vi "Agilent PWM Trigger and Fetch.vi"(7 "Agilent PWM":T1, 8 "error in (no error)":errorcluster, 10 "Timeout (10000ms)":u32=10000, 11 "VISA Resource Name":refnum<visa-resource-name>) -> (0 "error out":errorcluster, 2 "Data Reading":T2 caption="This reading is allways in the base units\ni.e. V, A, Ohms, Hz, Sec, dB, etc." format="%#_10f", 3 "dup VISA Resource Name":refnum<visa-resource-name>)   [LabVIEW 2011]
doc: "This VI for the HP 8753 is used to read the sweep type.\n\n0 LINEAR FREQ\n1 LOG FREQ\n2 LIST FREQ\n3 CW TIME\n4 POWER SWEEP"
uses:
  PWM Measurement.ctl
  TypeDefs/Agilent PWM Instrument Info.ctl
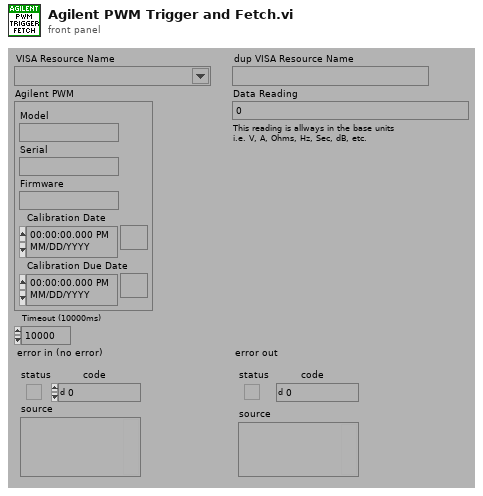
[diagram p1: front panel]
types:
  T1 = typedef "Agilent PWM Instrument Info.ctl" = cluster{"Model":string, "Serial":string, "Firmware":string, "Calibration Date":timestamp, "Calibration Due Date":timestamp}
  T2 = typedef "PWM Measurement.ctl" = dbl
  T3 = typedef "Agilent PWM Model.ctl" = enum16{"Not Supported", "E4418X", "E4419X", "U2000X"}
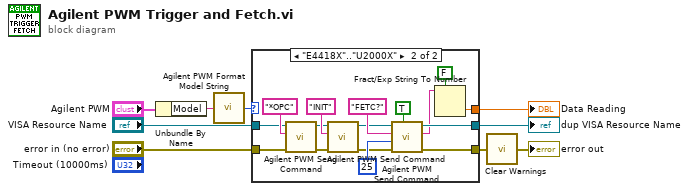
[diagram p0: block diagram]
diagram:
  n1 = Unbundle By Name("Agilent PWM") -> ("Model"=w3:string)
  n2 = call "Agilent PWM Format Model String.vi"("Model"=w3) -> ("Model"=w1:T3)
  n3 = case shown="\"E4418X\"..\"U2000X\"" w1 {
    tunnel: [_ w24] -> w9
    tunnel: "VISA Resource Name" -> [w11 w22]
    tunnel: "error in (no error)" -> [w10 w19]
    tunnel: [w11 w18] -> w5
    tunnel: [w10 w17] -> w4
    frame "Not Supported" {
    }
    frame "E4418X".."U2000X" {
      n4 = call "Agilent PWM Send Command.vi"("error in (no error)"=w19, "Command"="*OPC" ("write buffer"), "VISA Resource Name"=w22) -> ("error out"=w20:errorcluster, "dup VISA Resource Name"=w21:refnum<visa-resource-name>)  [unwired: 2 in, 5 out]
      n5 = call "Agilent PWM Send Command.vi"("error in (no error)"=w20, "Command"="INIT" ("write buffer"), "VISA Resource Name"=w21) -> ("error out"=w13:errorcluster, "dup VISA Resource Name"=w12:refnum<visa-resource-name>)  [unwired: 2 in, 5 out]
      n6 = call "Agilent PWM Send Command.vi"("Read? (F)"=TRUE, "error in (no error)"=w13, "Byte Count"=u32 25 ("byte count"), "Command"="FETC?" ("write buffer"), "VISA Resource Name"=w12) -> ("error out"=w17:errorcluster, "Data Read"=w16:string, "dup VISA Resource Name"=w18:refnum<visa-resource-name>)  [unwired: 4 out]
      n7 = Fract/Exp String To Number(use system decimal point (T)=FALSE, string=w16) -> (number=w24:dbl)  [unwired: 3 out]
    }
  }
  "dup VISA Resource Name" <- w5
  "Data Reading" <- w9
  n8 = call "Clear Warnings.vi"("error in (no error)"=w4) -> ("error out"=→"error out":errorcluster)
